vi "Pause Timer.vi"(8 "error in (no error)":errorcluster, 11 "Timer Demo App in":refnum<class "Timer Demo App.lvclass">) -> (0 "error out":errorcluster, 3 "Timer Demo App out":refnum<class "Timer Demo App.lvclass">)   [LabVIEW 2020, in "Timer Demo.lvlib" / "Timer Demo App.lvclass"]
uses:
  Timer Demo App.lvclass
  Timer Demo App.lvclass/Timer Demo App.ctl
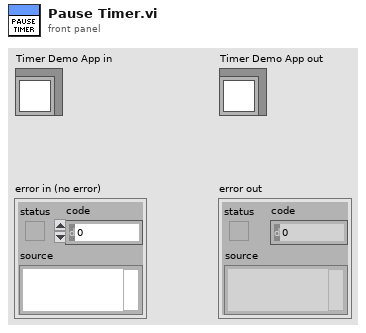
[diagram p1: front panel]
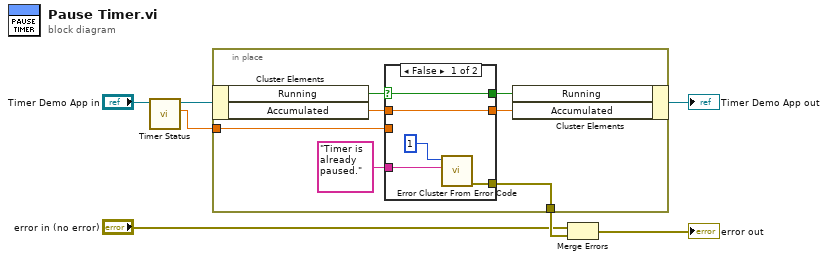
[diagram p0: block diagram]
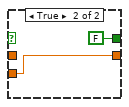
[diagram p2: hidden frame]
diagram:
  n1 = call "Timer Status.vi"("Timer Demo App in"="Timer Demo App in") -> ("Elapsed"=w1:dbl, "Timer Demo App out"=w2:refnum<class "Timer Demo App.lvclass">)  [unwired: 7 in, 2 out]
  n2 = in-place {
    in-place-border: [w11] -> w7
    in-place-border: w1 -> [w10]
    n3 = in-place-cluster #1(w2) -> ("Running"=w14:bool, "Accumulated"=w9:dbl)
    n4 = case shown="False" w14 {
      selector: w14 -> [w19 _]
      tunnel: [w19 FALSE] -> w13
      tunnel: "Timer is already paused." ("error message (\"\")") -> [w17 _]
      tunnel: [w16 _] -> w11
      tunnel: w10 -> [_ w20]
      tunnel: w9 -> [w15 _]
      tunnel: [w15 w20] -> w8
      frame False {
        n5 = call <vilib>:"Error Cluster From Error Code.vi"("error message (\"\")"=w17, "error code (0)"=1) -> ("error out"=w16:errorcluster)  [unwired: 7 in]
      }
      frame True {
      }
    }
    n6 = in-place-cluster #1("Running"=w13, "Accumulated"=w8) -> (→"Timer Demo App out":refnum<class "Timer Demo App.lvclass">)
  }
  n7 = Merge Errors("error in (no error)", w7) -> (→"error out":errorcluster)
